vi "ficherosubvi.vi"(8 "error in (no error)":errorcluster, 9 "Formato":string, 10 "Nombre del Archivo":string, 11 "Direccion":path) -> (0 "error out":errorcluster, 3 "Byte Stream File out":refnum<file>)   [LabVIEW 2020]
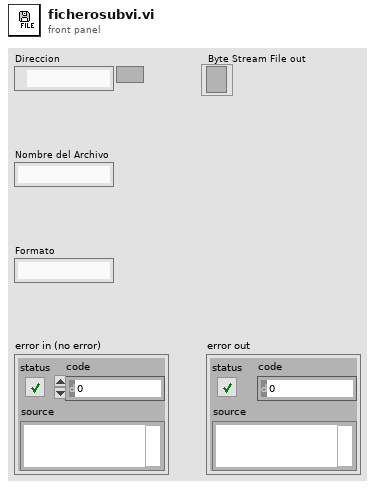
[diagram p1: front panel]
types:
  T1 = enum16{"open", "replace", "create", "open or create", "replace or create", "replace or create with confirmation"}
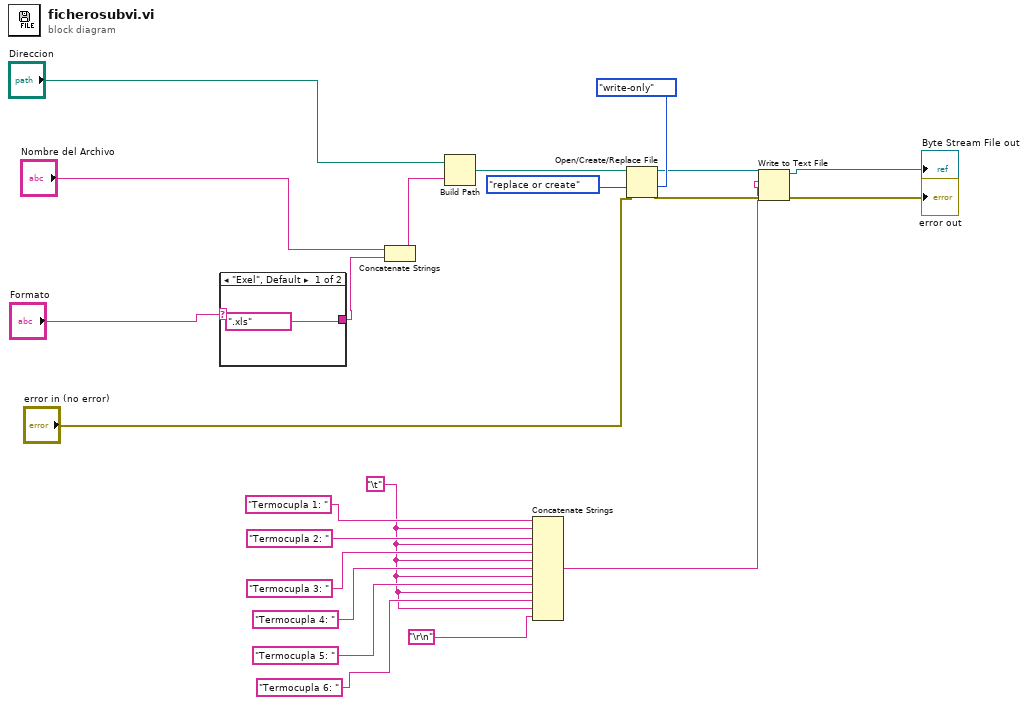
[diagram p0: block diagram]
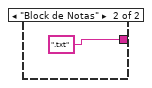
[diagram p2: hidden frame]
diagram:
  w3 = "\t"
  n1 = case shown="\"Exel\", Default" "Formato" {
    tunnel: [".xls" ".txt"] -> w17
    frame "Exel", Default {
    }
    frame "Block de Notas" {
    }
  }
  n2 = Concatenate Strings("Nombre del Archivo", w17) -> (w18:string)
  n3 = Build Path(base path="Direccion", name or relative path=w18) -> (appended path=w19:path)
  n4 = Concatenate Strings("Termocupla 1: ", w3, "Termocupla 2: ", w3, "Termocupla 3: ", w3, "Termocupla 4: ", w3, "Termocupla 5: ", w3, "Termocupla 6: ", w3, "\r\n") -> (w1:string)
  n5 = Open/Create/Replace File(file path (use dialog)=w19, error in="error in (no error)", operation (0:open)=T1."replace or create", access (0:read/write)=enum16{"read/write", "read-only", "write-only"}."write-only") -> (refnum out=w13:refnum<file>, error out=w12:errorcluster)  [unwired: 2 in, 1 out]
  n6 = Write to Text File(file (use dialog)=w13, text=w1, error in=w12) -> (refnum out=→"Byte Stream File out":refnum<file>, error out=→"error out":errorcluster)  [unwired: 1 in, 1 out]
